vi "Begin.vi"() -> (0 "error out":errorcluster)   [LabVIEW 2013]
doc: "Called before other user functions, this VI is expected to open initial I/O refnums, load in file data, and do all program initialization. Notice that the <B>error out</B> terminal is simply used for data flow. Wiring it to other structures or subVIs ensures that this VI runs first."
uses:
  <vilib>/Rock Robotics/WPI/Joystick/WPI_JoystickDeviceEnum.ctl
  <vilib>/Rock Robotics/SystemInterfaces/Typedef/FPGA_TypedefDigitalModule.ctl
  <vilib>/Rock Robotics/SystemInterfaces/Typedef/FPGA_TypedefSolenoidModule.ctl
  <vilib>/Rock Robotics/WPI/Solenoid/WPI_SolenoidChannel.ctl
  <vilib>/Rock Robotics/WPI/Solenoid/WPI_SolenoidValue.ctl
  <vilib>/Rock Robotics/WPI/Camera/WPI_CameraImageSize.ctl
  <vilib>/Rock Robotics/WPI/Camera/WPI_CameraWhite Balance Values.ctl
  <vilib>/Rock Robotics/WPI/Camera/WPI_CameraExposure Values.ctl
  <vilib>/Rock Robotics/WPI/Camera/WPI_CameraFrameRate.ctl
  <vilib>/Rock Robotics/SystemInterfaces/DIO/FPGA_DIOPWMChannel.ctl
  <vilib>/Rock Robotics/SystemInterfaces/DIO/FPGA_DIOChannel.ctl
  <vilib>/Rock Robotics/SystemInterfaces/DIO/FPGA_DIORelayChannel.ctl
  <vilib>/Rock Robotics/WPI/Solenoid/WPI_SolenoidOpenDouble.vi
  <vilib>/Rock Robotics/WPI/Solenoid/WPI_SolenoidSetEnum.vi
  <vilib>/Rock Robotics/WPI/RobotDrive/WPI_RobotDriveOpen2MotorWithVictor.vi
  <vilib>/Rock Robotics/WPI/Counter/WPI_CounterDigitalInputToDigitalSource.vi
  <vilib>/Rock Robotics/WPI/Compressor/WPI_CompressorGetSetRefNum.vi
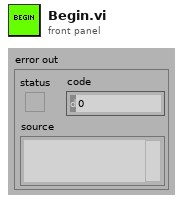
[diagram p1: front panel]
types:
  T1 = typedef "WPI_JoystickDeviceEnum.ctl" = enum16{"USB 1", "USB 2", "USB 3", "USB 4", "Kinect 1", "Kinect 2"}
  T2 = typedef "FPGA_TypedefDigitalModule.ctl" = enum16{"Digital Module 1", "Digital Module 2"}
  T3 = typedef "WPI_CameraDevRef.ctl" = cluster{"Camera Address":string, "CameraStatus":errorcluster, "Acquire Image Notifier":refnum<notifier>}
  T4 = typedef "WPI_CameraFrameRate.ctl" = u32
  T5 = typedef "WPI_CameraExposure Values.ctl" = enum16{"Auto", "Flicker-free 50 Hz", "Flicker-free 60 Hz", "Hold current"}
  T6 = typedef "WPI_CameraWhite Balance Values.ctl" = enum16{"Auto", "Fixed indoor", "Fixed outdoor 1", "Fixed outdoor 2", "Fixed fluorescent 1", "Fixed fluorescent 2", "Hold current"}
  T7 = typedef "WPI_CameraImageSize.ctl" = enum16{"640x480", "320x240", "160x120"}
  T8 = typedef "FPGA_DIOChannel.ctl" = enum8{"DIO 1", "DIO 2", "DIO 3", "DIO 4", "DIO 5", "DIO 6", "DIO 7", "DIO 8", "DIO 9", "DIO 10", "DIO 11", "DIO 12", "DIO 13", "DIO 14", "Invalid"}
  T9 = typedef "FPGA_DIOPWMChannel.ctl" = enum8{"PWM 1", "PWM 2", "PWM 3", "PWM 4", "PWM 5", "PWM 6", "PWM 7", "PWM 8", "PWM 9", "PWM 10", "Invalid"}
  T10 = typedef "WPI_DigitalInputDevRef.ctl" = cluster{"DevStatus":errorcluster, "DIO Channel":T8, "Digital Module":T2}
  T11 = typedef "WPI_RobotDriveDevRef.ctl" = cluster{"DevStatus":errorcluster, "Motors[]":T12[], "Square Inputs":bool, "Max Output":dbl, "Isochronous":bool}
  T12 = typedef "WPI_MotorControlDeviceRef.ctl" = cluster{"DeviceStatus":errorcluster, "Type":enum16{"PWM", "CAN"}, "PWM":cluster{"Digital Module":T2, "PWM Channel":T9, "DeadBand":T13}, "CAN":cluster{"Device Number":u8, "Control Mode":T14, "Semaphore":T15, "Max Vout":dbl}, "Invert":bool, "TransformRef":T16, "InvTransformRef":T16}
  T13 = typedef "WPI_PWMDeadband.ctl" = cluster{"Name":string, "maxPositivePwm":i32, "minPositivePwm":i32, "centerPwm":i32, "maxNegativePwm":i32, "minNegativePwm":i32, "angularRange":u16}
  T14 = typedef "WPI_CANJaguar_ControlMode.ctl" = enum8{"Percent VBus", "Current", "Speed", "Position", "Voltage"}
  T15 = typedef "Semaphore RefNum" = refnum<k1>
  T16 = typedef "WPI_PWMTransform_ConPane.ctl" = refnum<vi>
  T17 = typedef "FPGA_CounterEncoderSourceConvertionLVSourceType.ctl" = cluster{"DevStatus":errorcluster, "AnalogTriggerMode?":bool, "DigitalMode":cluster{"Digital Module":T2, "DIO Channel":T18}, "AnalogTriggerMode":cluster{"AnalogTriggerIndex":T19, "OutputType":T20}}
  T18 = typedef "FPGA_DIODigitalSourceChannel.ctl" = enum8{"DIO 1", "DIO 2", "DIO 3", "DIO 4", "DIO 5", "DIO 6", "DIO 7", "DIO 8", "DIO 9", "DIO 10", "DIO 11", "DIO 12", "DIO 13", "DIO 14", "Disabled"}
  T19 = typedef "FPGA_AnalogTriggerIndex.ctl" = enum8{"Trig 0", "Trig 1", "Trig 2", "Trig 3", "Trig 4", "Trig 5", "Trig 6", "Trig 7", "Invalid"}
  T20 = typedef "FPGA_AnalogTriggerOutType.ctl" = enum16{"InWindow", "TriggerState", "Rising", "Falling"}
  T21 = typedef "WPI_EncoderDevRef.ctl" = cluster{"DevStatus":errorcluster, "EncoderIndex":T22, "CounterIndex":T23, "DistancePerCount":dbl, "Decoding Type":T24}
  T22 = typedef "FPGA_EncoderIdx.ctl" = enum8{"Enc 0", "Enc 1", "Enc 2", "Enc 3", "Invalid"}
  T23 = typedef "FPGA_CounterCtrSystemIndex.ctl" = enum8{"Ctr 0", "Ctr 1", "Ctr 2", "Ctr 3", "Ctr 4", "Ctr 5", "Ctr 6", "Ctr 7", "Invalid"}
  T24 = typedef "WPI_EncoderType.ctl" = enum16{"1x", "2x", "4x"}
  T25 = typedef "WPI_SolenoidValue.ctl" = enum16{"Off", "On", "Forward", "Reverse"}
  T26 = typedef "WPI_SolenoidChannel.ctl" = enum8{"Solenoid 1", "Solenoid 2", "Solenoid 3", "Solenoid 4", "Solenoid 5", "Solenoid 6", "Solenoid 7", "Solenoid 8", "Invalid"}
  T27 = typedef "FPGA_TypedefSolenoidModule.ctl" = enum16{"Solenoid Module 1", "Solenoid Module 2"}
  T28 = typedef "WPI_SolenoidDevRef.ctl" = cluster{"DevStatus":errorcluster, "Solenoid Module":T27, "Forward Solenoid Channel":T26, "Reverse Solenoid Channel":T26}
  T29 = typedef "FPGA_DIORelayChannel.ctl" = enum8{"Relay 1", "Relay 2", "Relay 3", "Relay 4", "Relay 5", "Relay 6", "Relay 7", "Relay 8", "Invalid"}
  T30 = typedef "WPI_CompressorDevRef.ctl" = cluster{"DevStatus":errorcluster, "DigitalInputDevRef":T10, "RelayDevRef":T31}
  T31 = typedef "WPI_RelayDevRef.ctl" = cluster{"DevStatus":errorcluster, "Relay Channel":T29, "Digital Module":T2, "Relay Direction":T32}
  T32 = typedef "WPI_RelayDirection.ctl" = enum16{"Both directions", "Forward only", "Reverse only"}
  T33 = typedef "WPI_JoystickDevRef.ctl" = cluster{"Device":T1}
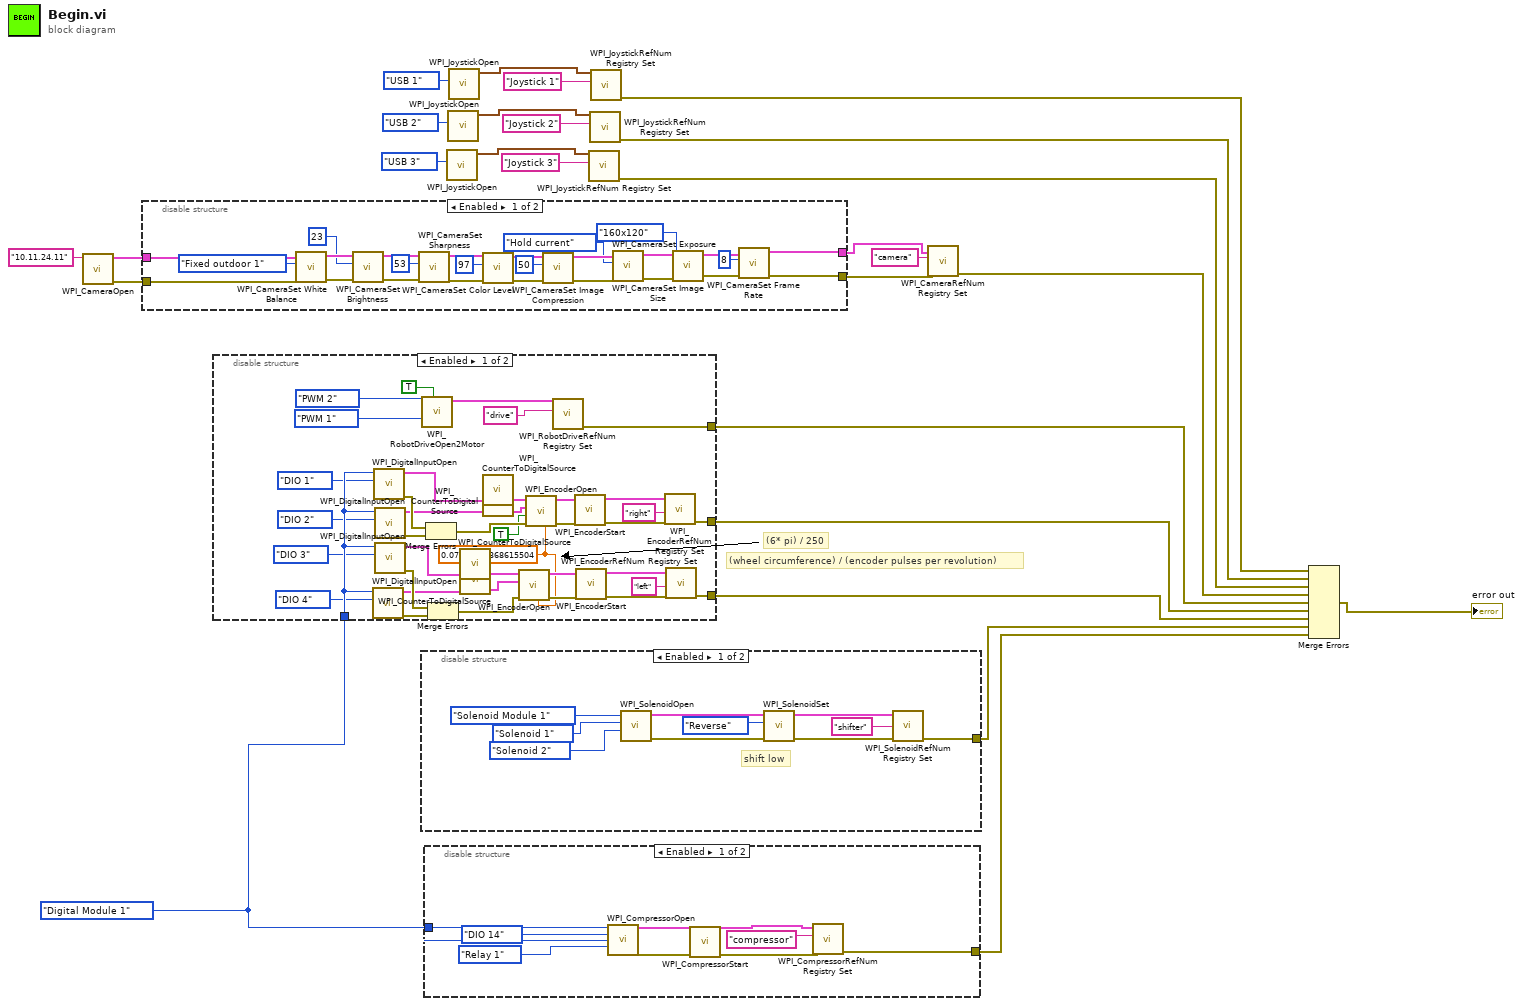
[diagram p0: block diagram]
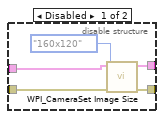
[diagram p6: hidden frame]
diagram:
  w10 = FPGA_TypedefDigitalModule."Digital Module 1" ("Digital Module (Module 1)")
  # "(wheel circumference) / (encoder pulses per revolution)"
  # "(6* pi) / 250"
  n1 = call <vilib>:"WPI_CameraOpen.vi"("Camera Address"="10.11.24.11") -> ("error out"=w2:errorcluster, "CameraDevRef"=w4:T3)  [unwired: 9 in]
  n2 = disable-structure shown="Enabled" {
    disable-tunnel: w4 -> [w50 w54]
    disable-tunnel: [w28 w53] -> w3
    disable-tunnel: w2 -> [w37 w56]
    disable-tunnel: [w27 w55] -> w1
    frame Enabled {
      n3 = call <vilib>:"WPI_CameraSet White Balance.vi"("error in (no error)"=w37, "White Balance"=WPI_CameraWhite_Balance_Values."Fixed outdoor 1", "CameraDevRef"=w50) -> ("error out"=w38:errorcluster, "CameraDevRef Out"=w49:T3)  [unwired: 7 in]
      n4 = call <vilib>:"WPI_CameraSet Brightness.vi"("error in (no error)"=w38, "Brightness"=23, "CameraDevRef"=w49) -> ("error out"=w39:errorcluster, "CameraDevRef Out"=w48:T3)  [unwired: 7 in]
      n5 = call <vilib>:"WPI_CameraSet Sharpness.vi"("error in (no error)"=w39, "Sharpness"=53, "CameraDevRef"=w48) -> ("error out"=w40:errorcluster, "CameraDevRef Out"=w47:T3)  [unwired: 7 in]
      n6 = call <vilib>:"WPI_CameraSet Color Level.vi"("error in (no error)"=w40, "Color Level"=97, "CameraDevRef"=w47) -> ("error out"=w41:errorcluster, "CameraDevRef Out"=w46:T3)  [unwired: 7 in]
      n7 = call <vilib>:"WPI_CameraSet Image Compression.vi"("error in (no error)"=w41, "Compression"=50, "CameraDevRef"=w46) -> ("error out"=w52:errorcluster, "CameraDevRef Out"=w51:T3)  [unwired: 7 in]
      n8 = call <vilib>:"WPI_CameraSet Exposure.vi"("error in (no error)"=w52, "Exposure"=WPI_CameraExposure_Values."Hold current", "CameraDevRef"=w51) -> ("error out"=w42:errorcluster, "CameraDevRef Out"=w45:T3)  [unwired: 7 in]
      n9 = call <vilib>:"WPI_CameraSet Image Size.vi"("error in (no error)"=w42, "Image Size"=WPI_CameraImageSize."160x120", "CameraDevRef"=w45) -> ("error out"=w43:errorcluster, "CameraDevRef Out"=w44:T3)  [unwired: 7 in]
      n10 = call <vilib>:"WPI_CameraSet Frame Rate.vi"("error in (no error)"=w43, "Frame Rate (fps)"=T4 8, "CameraDevRef"=w44) -> ("error out"=w27:errorcluster, "CameraDevRef Out"=w28:T3)  [unwired: 7 in]
    }
    frame Disabled {
      n11 = disable-structure shown="Enabled" {
        disable-tunnel: w56 -> [w60 w62]
        disable-tunnel: [w59 w62] -> w55
        disable-tunnel: w54 -> [w58 w63]
        disable-tunnel: [w57 w63] -> w53
        frame Disabled {
          n12 = call <vilib>:"WPI_CameraSet Image Size.vi"("error in (no error)"=w60, "Image Size"=WPI_CameraImageSize."160x120", "CameraDevRef"=w58) -> ("error out"=w59:errorcluster, "CameraDevRef Out"=w57:T3)  [unwired: 7 in]
        }
        frame Enabled {
        }
      }
    }
  }
  n13 = disable-structure shown="Enabled" {
    disable-tunnel: w10 -> [w82 _]
    disable-tunnel: [w76 _] -> w13
    disable-tunnel: [w75 _] -> w12
    disable-tunnel: [w74 _] -> w11
    frame Enabled {
      w77 = 0.07539822368615504 ("DistancePerCount")
      n14 = call <vilib>:"WPI_DigitalInputOpen.vi"("DIO Channel"=FPGA_DIOChannel."DIO 4", "Digital Module (Module 1)"=w82) -> ("error out"=w73:errorcluster, "DigitalInputDevRef"=w66:T10)  [unwired: 8 in]
      n15 = call <vilib>:"WPI_DigitalInputOpen.vi"("DIO Channel"=FPGA_DIOChannel."DIO 1", "Digital Module (Module 1)"=w82) -> ("error out"=w68:errorcluster, "DigitalInputDevRef"=w86:T10)  [unwired: 8 in]
      n16 = call <vilib>:"WPI_DigitalInputOpen.vi"("DIO Channel"=FPGA_DIOChannel."DIO 2", "Digital Module (Module 1)"=w82) -> ("error out"=w70:errorcluster, "DigitalInputDevRef"=w67:T10)  [unwired: 8 in]
      n17 = call <vilib>:"WPI_DigitalInputOpen.vi"("DIO Channel"=FPGA_DIOChannel."DIO 3", "Digital Module (Module 1)"=w82) -> ("error out"=w71:errorcluster, "DigitalInputDevRef"=w100:T10)  [unwired: 8 in]
      n18 = call-poly <vilib>:"WPI_RobotDriveOpen2Motor.vi"("Left Motor Inverted"=TRUE, "Right Motor"=FPGA_DIOPWMChannel."PWM 1", "Left Motor"=FPGA_DIOPWMChannel."PWM 2") -> ("RobotDriveDevRef"=w102:T11)  [unwired: 7 in, 1 out]
      n19 = Merge Errors(w68, w70) -> (w69:errorcluster)
      n20 = Merge Errors(w71, w73) -> (w72:errorcluster)
      n21 = call-poly <vilib>:"WPI_CounterToDigitalSource.vi"("DigitalInputDevRef"=w100) -> ("Digital Source"=w93:T17)  [unwired: 6 in]
      n22 = call-poly <vilib>:"WPI_CounterToDigitalSource.vi"("DigitalInputDevRef"=w66) -> ("Digital Source"=w94:T17)  [unwired: 6 in]
      n23 = call-poly <vilib>:"WPI_CounterToDigitalSource.vi"("DigitalInputDevRef"=w86) -> ("Digital Source"=w92:T17)  [unwired: 6 in]
      n24 = call-poly <vilib>:"WPI_CounterToDigitalSource.vi"("DigitalInputDevRef"=w67) -> ("Digital Source"=w91:T17)  [unwired: 6 in]
      n25 = call <vilib>:"WPI_EncoderOpen.vi"("DistancePerCount"=w77, "error in (no error)"=w72, "BSource"=w94, "ASource"=w93) -> ("error out"=w95:errorcluster, "EncoderDevRef"=w96:T21)  [unwired: 6 in]
      n26 = call <vilib>:"WPI_EncoderOpen.vi"("DistancePerCount"=w77, "error in (no error)"=w69, "Invert Direction (False)"=TRUE, "BSource"=w91, "ASource"=w92) -> ("error out"=w90:errorcluster, "EncoderDevRef"=w89:T21)  [unwired: 5 in]
      n27 = call <vilib>:"WPI_RobotDriveRefNum Registry Set.vi"("refnum name"="drive", "RobotDriveDevRef"=w102) -> ("error out"=w76:errorcluster)  [unwired: 8 in, 1 out]
      n28 = call <vilib>:"WPI_EncoderStart.vi"("error in (no error)"=w90, "EncoderDevRef"=w89) -> ("error out"=w88:errorcluster, "EncoderDevRef"=w87:T21)  [unwired: 8 in]
      n29 = call <vilib>:"WPI_EncoderStart.vi"("error in (no error)"=w95, "EncoderDevRef"=w96) -> ("error out"=w97:errorcluster, "EncoderDevRef"=w98:T21)  [unwired: 8 in]
      n30 = call <vilib>:"WPI_EncoderRefNum Registry Set.vi"("error in (no error)"=w88, "refnum name"="right", "EncoderDevRef"=w87) -> ("error out"=w75:errorcluster)  [unwired: 7 in, 1 out]
      n31 = call <vilib>:"WPI_EncoderRefNum Registry Set.vi"("error in (no error)"=w97, "refnum name"="left", "EncoderDevRef"=w98) -> ("error out"=w74:errorcluster)  [unwired: 7 in, 1 out]
    }
    frame Disabled {
    }
  }
  n32 = disable-structure shown="Enabled" {
    disable-tunnel: [w108 _] -> w9
    frame Enabled {
      # "shift low"
      n33 = call-poly <vilib>:"WPI_SolenoidOpen.vi"("Reverse Solenoid Channel"=WPI_SolenoidChannel."Solenoid 2", "Forward Solenoid Channel"=WPI_SolenoidChannel."Solenoid 1", "Solenoid Module (Module 1)"=FPGA_TypedefSolenoidModule."Solenoid Module 1") -> ("error out"=w105:errorcluster, "SolenoidDevRef"=w106:T28)  [unwired: 7 in]
      n34 = call-poly <vilib>:"WPI_SolenoidSet.vi"("error in (no error)"=w105, "Value"=WPI_SolenoidValue."Reverse", "SolenoidDevRef"=w106) -> ("error out"=w104:errorcluster, "SolenoidDevRef"=w103:T28)  [unwired: 7 in]
      n35 = call <vilib>:"WPI_SolenoidRefNum Registry Set.vi"("error in (no error)"=w104, "refnum name"="shifter", "SolenoidDevRef"=w103) -> ("error out"=w108:errorcluster)  [unwired: 7 in, 1 out]
    }
    frame Disabled {
    }
  }
  n36 = disable-structure shown="Enabled" {
    disable-tunnel: w10 -> [w120 _]
    disable-tunnel: [w117 _] -> w8
    frame Enabled {
      n37 = call <vilib>:"WPI_CompressorOpen.vi"("Pressure Switch Digital Module (Module 1)"=w120, "Pressure Switch DIO Channel"=FPGA_DIOChannel."DIO 14", "Relay Digital Module (Module 1)"=w120, "Relay Channel"=FPGA_DIORelayChannel."Relay 1") -> ("CompressorDevRef"=w116:T30, "error out"=w115:errorcluster)  [unwired: 10 in]
      n38 = call <vilib>:"WPI_CompressorStart.vi"("error in (no error)"=w115, "CompressorDevRef"=w116) -> ("error out"=w114:errorcluster, "CompressorDevRef"=w113:T30)  [unwired: 8 in]
      n39 = call <vilib>:"WPI_CompressorRefNum Registry Set.vi"("error in (no error)"=w114, "refnum name"="compressor", "CompressorDevRef"=w113) -> ("error out"=w117:errorcluster)  [unwired: 7 in, 1 out]
    }
    frame Disabled {
    }
  }
  n40 = call <vilib>:"WPI_JoystickOpen.vi"("JoystickDevice"=WPI_JoystickDeviceEnum."USB 3") -> ("JoystickDevRef"=w25:T33)  [unwired: 10 in]
  n41 = call <vilib>:"WPI_JoystickOpen.vi"("JoystickDevice"=WPI_JoystickDeviceEnum."USB 2") -> ("JoystickDevRef"=w22:T33)  [unwired: 10 in]
  n42 = call <vilib>:"WPI_JoystickOpen.vi"("JoystickDevice"=WPI_JoystickDeviceEnum."USB 1") -> ("JoystickDevRef"=w19:T33)  [unwired: 10 in]
  n43 = call <vilib>:"WPI_JoystickRefNum Registry Set.vi"("refnum name"="Joystick 3", "JoystickDevRef"=w25) -> ("error out"=w15:errorcluster)  [unwired: 8 in, 1 out]
  n44 = call <vilib>:"WPI_JoystickRefNum Registry Set.vi"("refnum name"="Joystick 2", "JoystickDevRef"=w22) -> ("error out"=w16:errorcluster)  [unwired: 8 in, 1 out]
  n45 = call <vilib>:"WPI_JoystickRefNum Registry Set.vi"("refnum name"="Joystick 1", "JoystickDevRef"=w19) -> ("error out"=w17:errorcluster)  [unwired: 8 in, 1 out]
  n46 = call <vilib>:"WPI_CameraRefNum Registry Set.vi"("error in (no error)"=w1, "refnum name"="camera", "CameraDevRef"=w3) -> ("error out"=w14:errorcluster)  [unwired: 7 in, 1 out]
  n47 = Merge Errors(w17, w16, w15, w14, w13, w12, w11, w9, w8) -> (→"error out":errorcluster)
